vi "FTW-Test-JSON-ObjectKeys.vi"() -> ()   [LabVIEW 2013]
uses:
  source/JSON/FTW-JSON.lvclass
  DRAP_SLASD-Core_LoadConfig Folder/Jobs/06520 DRAP/06310 DRAP/source/System Launcher and Service Directory/Core/DRAP_SLASD-Core_Device.ctl
panel:
  in  "Logger Address":string
  out "Devices":T1[](array[typedef])
  out "System Launcher Configuration":string
  in  "error in":errorcluster
  out "error out":errorcluster
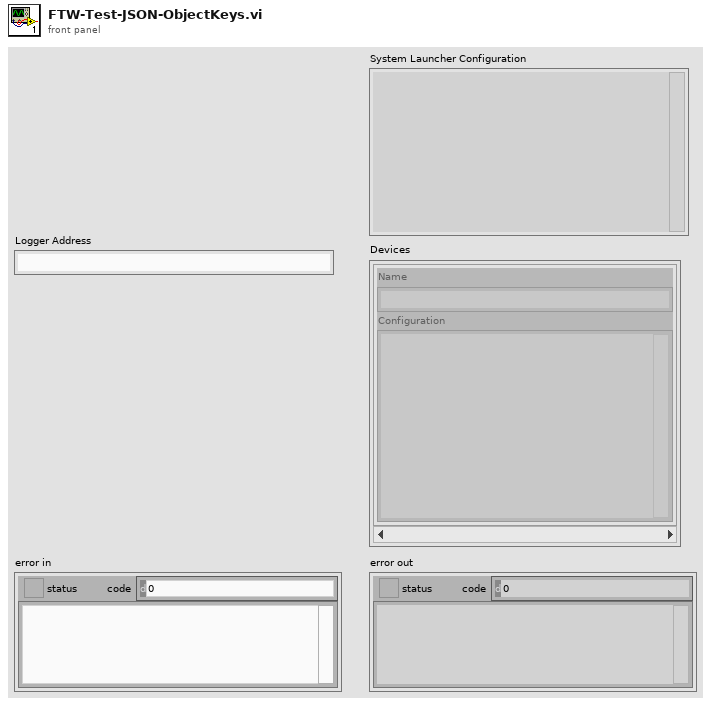
[diagram p1: front panel]
types:
  T1 = typedef "DRAP_SLASD-Core_Device.ctl" = cluster{"Name":string, "Configuration":string}
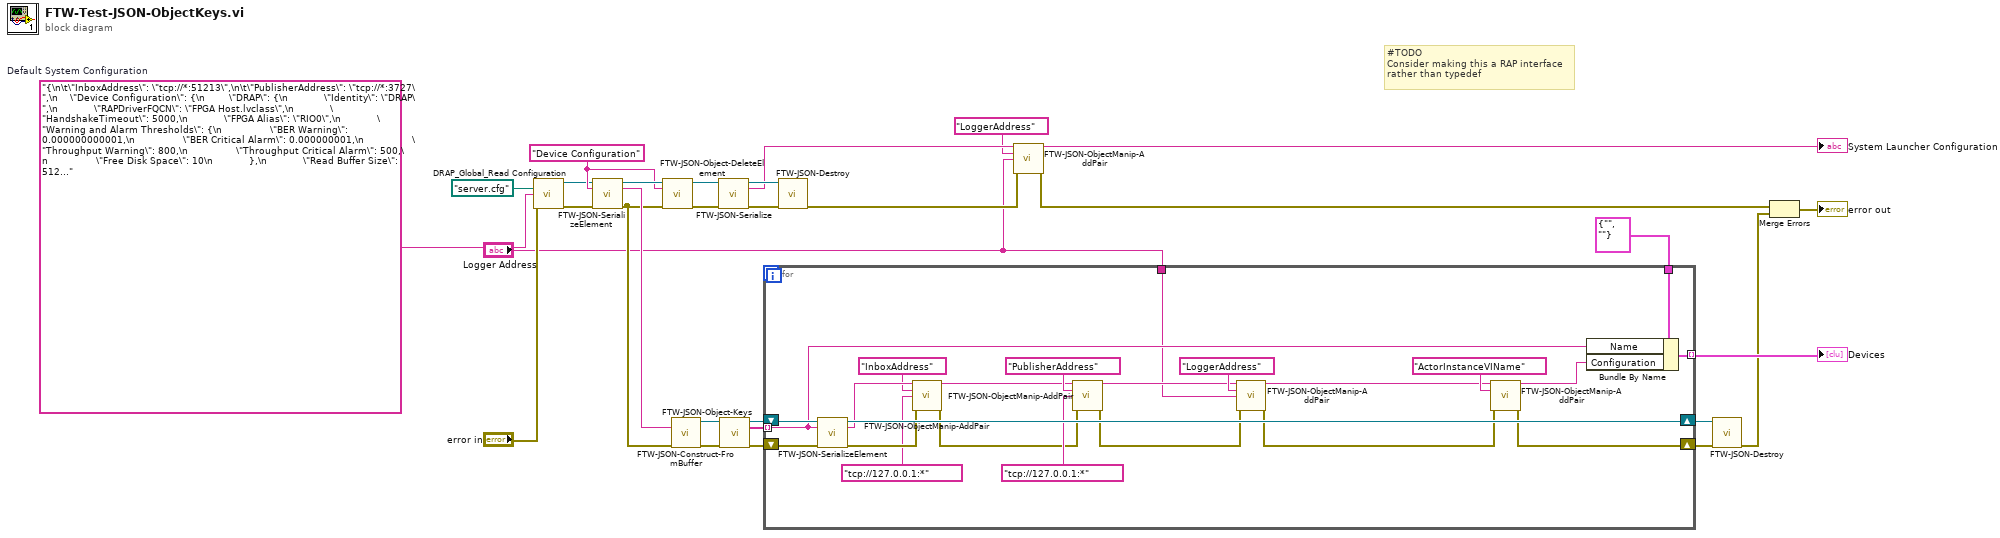
[diagram p0: block diagram]
diagram:
  w29 = "Device Configuration" ("Key")
  w7 = "{\n\t\"InboxAddress\": \"tcp://*:51213\",\n\t\"PublisherAddress\": \"tcp://*:3727\",\n    \"Device Configuration\": {\n        \"DRAP\": {\n            \"Identity\": \"DRAP\",\n            \"RAPDriverFQCN\": \"FPGA Host.lvclass\",\n            \"HandshakeTimeout\": 5000,\n            \"FPGA Alias\": \"RIO0\",\n            \"Warning and Alarm Thresholds\": {\n                \"BER Warning\": 0.000000000001,\n                \"BER Critical Alarm\": 0.000000001,\n                \"Throughput Warning\": 800,\n                \"Throughput Critical Alarm\": 500,\n                \"Free Disk Space\": 10\n            },\n            \"Read Buffer Size\": 512,\n            \"Write Buffer Size\": 512,\n            \"Throughput/BER Calculation Period\": 200,\n            \"LoopPeriod\": 50\n        }\n    }\n}"  # Default System Configuration
  # "#TODO\nConsider making this a RAP interface\nrather than typedef"
  n1 = call "DRAP_Global_Read Configuration.vi"("Configuration File"=path "server.cfg", "Default Configuration"=w7, "error in"="error in") -> ("Configuration"=w10:refnum<class "FTW-JSON.lvclass">, "error out"=w8:errorcluster)  [unwired: 10 in, 1 out]
  n2 = call "FTW-JSON-SerializeElement.vi"("JSON Object"=w10, "Key"=w29, "error in"=w8) -> ("JSON Object"=w30:refnum<class "FTW-JSON.lvclass">, "Element as JSON String"=w24:string, "error out"=w23:errorcluster)  [unwired: 9 in, 1 out]
  n3 = call "FTW-JSON-Object-DeleteElement.vi"("JSON Object"=w30, "Key"=w29, "error in"=w23) -> ("JSON Object out"=w28:refnum<class "FTW-JSON.lvclass">, "error out"=w27:errorcluster)  [unwired: 10 in, 1 out]
  n4 = call "FTW-JSON-Construct-FromBuffer.vi"("JSON String (UTF-8)"=w24, "error in"=w23) -> ("JSON Object"=w22:refnum<class "FTW-JSON.lvclass">, "error out"=w21:errorcluster)  [unwired: 12 in]
  n5 = call "FTW-JSON-Serialize.vi"("JSON Object"=w28, "error in"=w27) -> ("JSON Object out"=w26:refnum<class "FTW-JSON.lvclass">, "JSON String (UTF-8)"=w6:string, "error out"=w25:errorcluster)  [unwired: 11 in]
  n6 = call "FTW-JSON-Object-Keys.vi"("JSON Object"=w22, "error in"=w21) -> ("JSON Object out"=w20:refnum<class "FTW-JSON.lvclass">, "Keys"=w18:string[], "error out"=w19:errorcluster)  [unwired: 10 in, 1 out]
  n7 = for {
    shift-right: [w51] -> w15
    shift-left: w20 -> [w54]
    tunnel: w18 -> [w49] mode=indexing
    tunnel: [w50] -> w17 mode=indexing
    tunnel: T1 {"Name"="", "Configuration"=""} ("Device") -> [w52]
    shift-right: [w38] -> w14
    shift-left: w19 -> [w53]
    tunnel: "Logger Address" -> [w32]
    n8 = call "FTW-JSON-SerializeElement.vi"("JSON Object"=w54, "Key"=w49, "error in"=w53) -> ("JSON Object"=w51:refnum<class "FTW-JSON.lvclass">, "Element as JSON String"=w48:string, "error out"=w47:errorcluster)  [unwired: 9 in, 1 out]
    n9 = call "FTW-JSON-ObjectManip-AddPair.vi"("Input JSON Object"=w48, "Key"="InboxAddress", "Value"="tcp://127.0.0.1:*", "error in"=w47) -> ("Output JSON Object"=w42:string, "error out"=w41:errorcluster)  [unwired: 10 in]
    n10 = call "FTW-JSON-ObjectManip-AddPair.vi"("Input JSON Object"=w42, "Key"="PublisherAddress", "Value"="tcp://127.0.0.1:*", "error in"=w41) -> ("Output JSON Object"=w35:string, "error out"=w33:errorcluster)  [unwired: 10 in]
    n11 = call "FTW-JSON-ObjectManip-AddPair.vi"("Input JSON Object"=w35, "Key"="LoggerAddress", "Value"=w32, "error in"=w33) -> ("Output JSON Object"=w34:string, "error out"=w31:errorcluster)  [unwired: 10 in]
    n12 = call "FTW-JSON-ObjectManip-AddPair.vi"("Input JSON Object"=w34, "Key"="ActorInstanceVIName", "error in"=w31) -> ("Output JSON Object"=w39:string, "Value"=w37:string, "error out"=w38:errorcluster)  [unwired: 10 in]
    n13 = Bundle By Name(cluster=w52, "Name"=w49, "Configuration"=w39) -> (w50:T1)
  }
  "Devices" <- w17
  n14 = call "FTW-JSON-Destroy.vi"("JSON Object"=w26, "error in"=w25) -> ("error out"=w3:errorcluster)  [unwired: 13 in]
  n15 = call "FTW-JSON-ObjectManip-AddPair.vi"("Input JSON Object"=w6, "Key"="LoggerAddress", "Value"="Logger Address", "error in"=w3) -> ("Output JSON Object"=→"System Launcher Configuration":string, "error out"=w2:errorcluster)  [unwired: 10 in]
  n16 = call "FTW-JSON-Destroy.vi"("JSON Object"=w15, "error in"=w14) -> ("error out"=w13:errorcluster)  [unwired: 13 in]
  n17 = Merge Errors(w2, w13) -> (→"error out":errorcluster)
